vi "Create.vi"(8 "error in (no error)":errorcluster) -> (0 "error out":errorcluster, 2 "Event Reg":refnum<event-registration>, 3 "Build Events API out":refnum<class "Build Events API.lvclass">)   [LabVIEW 2020, in "Builder Tools.lvlib" / "Build Events API.lvclass"]
uses:
  Build Events API.lvclass
  Build Events API.lvclass/Build Events API.ctl
  Builder Tools.lvlib
  Enable Cancel Data.ctl
  New Job Data.ctl
  New Item Data.ctl
  Complete Data.ctl
  Error Data.ctl
  Build Events.ctl
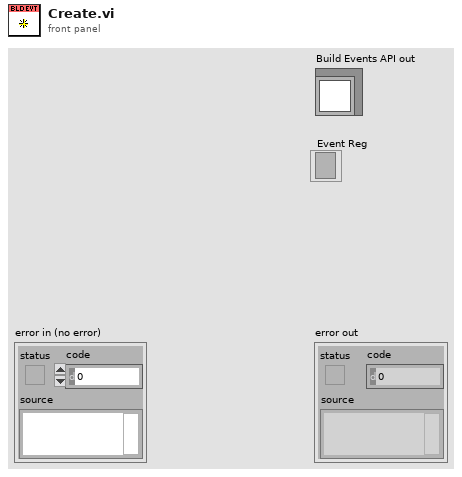
[diagram p1: front panel]
types:
  T1 = typedef "Builder Tools.lvlib/Build Events.ctl" = cluster{"Enable Cancel":refnum<user-event>, "New Job":refnum<user-event>, "New Item":refnum<user-event>, "Complete":refnum<user-event>, "Error":refnum<user-event>}
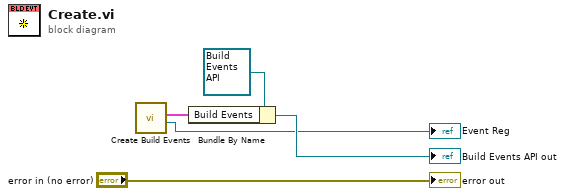
[diagram p0: block diagram]
diagram:
  n1 = call "Create Build Events.vi"() -> ("Event Reg"=→"Event Reg":refnum<event-registration>, "Build Events"=w2:T1)  [unwired: 10 in]
  n2 = Bundle By Name(cluster=refnum<class "Build Events API.lvclass"> refnum ("Build Events API in"), "Build Events"=w2) -> (→"Build Events API out":refnum<class "Build Events API.lvclass">)
  "error out" <- "error in (no error)"
